vi "RemoveDuplicates_D.vi"(11 "1D Array In":dbl[](array[numeric])) -> (3 "1D Array Out":dbl[](array[numeric]))   [LabVIEW 2009]
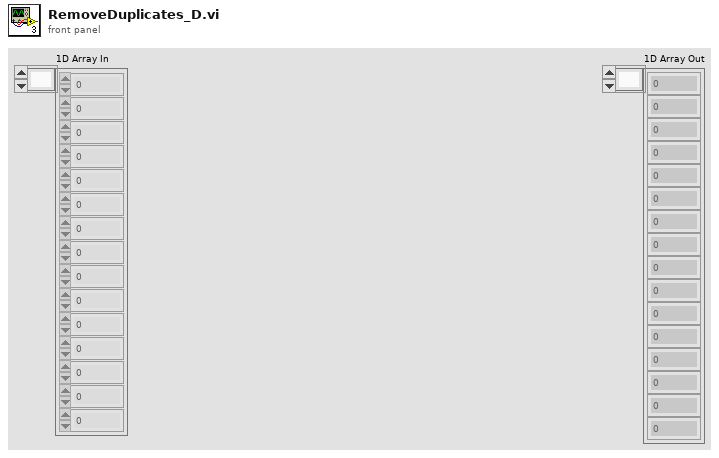
[diagram p1: front panel]
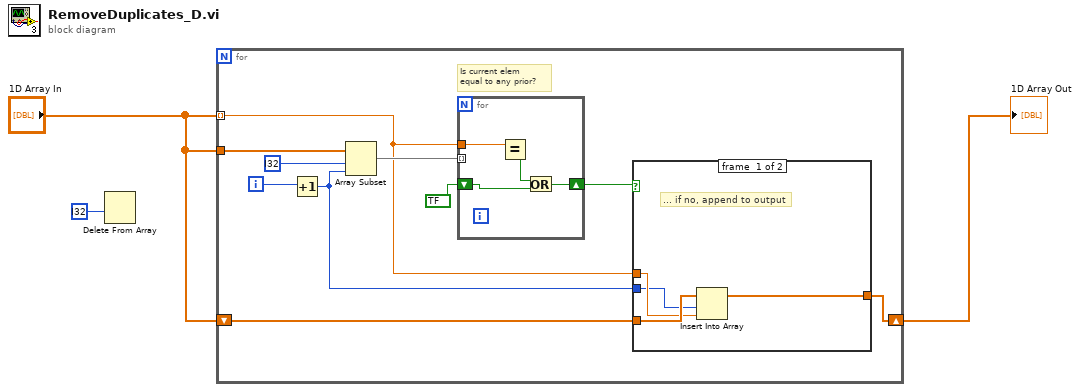
[diagram p0: block diagram]
diagram:
  n1 = Delete From Array(length=i32 ?) -> ()  [unwired: 2 in, 2 out]
  n2 = for {
    shift-right: [w5] -> w2
    shift-left: "1D Array In" -> [w6]
    tunnel: "1D Array In" -> [w7] mode=indexing
    tunnel: "1D Array In" -> [w4]
    i -> [w12]
    # "Is current elem\nequal to any prior?"
    n3 = Increment(x=w12) -> (x+1=w8:i32)
    n4 = Array Subset(array=w4, index=i32 ?, length=w8) -> (w11:dbl[])
    n5 = for {
      tunnel: w11 -> [_] mode=indexing
      tunnel: w7 -> [w22]
      shift-right: [w20] -> w9
      shift-left: bool ? -> [w19]
      n6 = Equal?(x=w22) -> (x = y?=w21:bool)  [unwired: 1 in]
      n7 = Or(x=w21, y=w19) -> (x .or. y?=w20:bool)
    }
    n8 = case shown="True" w9 {
      tunnel: w8 -> [w14 _]
      tunnel: w7 -> [w15 _]
      tunnel: w6 -> [w17 w18]
      tunnel: [w16 w18] -> w5
      frame #0 {
        # "... if no, append to output"
        n9 = Insert Into Array(array=w17, index=w14, new element=w15) -> (w16:dbl[])
      }
      frame #1 {
        # "... if yes, pass through"
      }
    }
  }
  "1D Array Out" <- w2
